vi "List Subscriptions.vi"(7 "Region":T1, 8 "error in (no error)":errorcluster, 11 "AWS Credentials":T2) -> (0 "error out":errorcluster, 3 "Subscriptions out":refnum<class "Subscription.lvclass">[](array[class]))   [LabVIEW 2015, in "NI_AWS_SNS.lvlib" / "Subscription.lvclass"]
uses:
  Subscription.lvclass
  Core/HTTP Request/AWS Credentials.ctl
  Core/HTTP Request/Region.ctl
  Core/HTTP Request/HTTP Request.lvclass/HTTP Request.ctl
  Core/HTTP Request/Write Credentials.vi
  Core/HTTP Request/Write Region.vi
  Core/HTTP Request/Write Service.vi
  Core/HTTP Request/Write Verify Server.vi
  Core/ARN/ARN.lvclass
  Core/HTTP Request/HTTP Request.lvclass
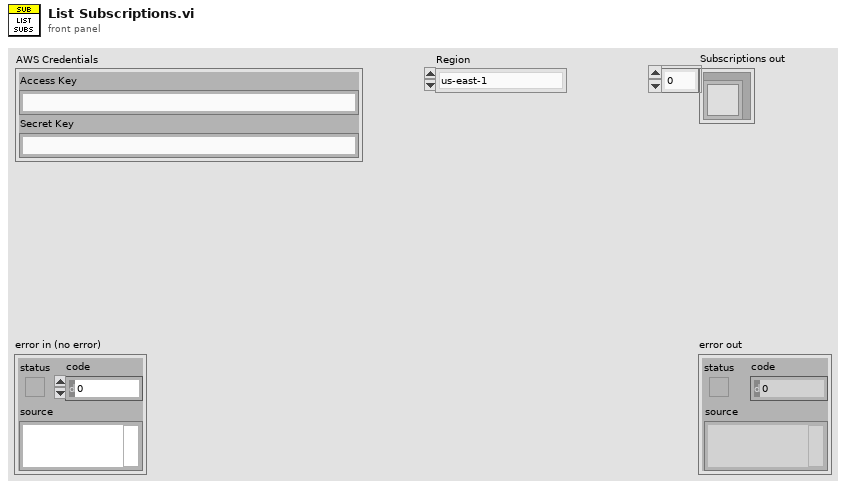
[diagram p1: front panel]
types:
  T1 = typedef "NI_AWS_Core.lvlib/HTTP Request.lvclass/Region.ctl" = enum16{"us-east-1", "us-east-2", "us-west-1", "us-west-2", "ap-northeast-1", "ap-northeast-2", "ap-southeast-1", "ap-southeast-2", "ca-central-1", "eu-central-1", "eu-west-1", "eu-west-2", "sa-east-1"}
  T2 = typedef "NI_AWS_Core.lvlib/HTTP Request.lvclass/AWS Credentials.ctl" = cluster{"Access Key":string, "Secret Key":string}
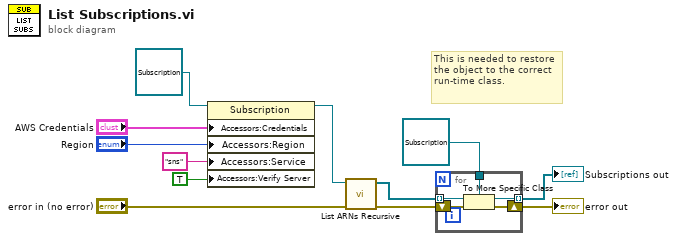
[diagram p0: block diagram]
diagram:
  # "This is needed to restore the object to the correct run-time class."
  n1 = property class="Subscription"(reference=refnum<class "Subscription.lvclass"> refnum ("NI_AWS_SNS.lvlib:Subscription"), "Accessors:Credentials"="AWS Credentials", "Accessors:Region"="Region", "Accessors:Service"="sns" ("Service"), "Accessors:Verify Server"=TRUE ("Verify Server")) -> (reference out=w10:refnum<class "Subscription.lvclass">)  [unwired: 1 in, 1 out]
  n2 = call "List ARNs Recursive.vi"("error in (no error)"="error in (no error)", "ARN in"=w10) -> ("error out"=w6:errorcluster, "ARNs out"=w8:refnum<class "ARN.lvclass">[])  [unwired: 8 in]
  n3 = for {
    tunnel: refnum<class "Subscription.lvclass"> refnum ("NI_AWS_SNS.lvlib:Subscription") -> [w17]
    tunnel: w8 -> [w16] mode=indexing
    tunnel: [w15] -> w4 mode=indexing
    shift-right: [w13] -> w1
    shift-left: w6 -> [w14]
    n4 = To More Specific Class(target class=w17, reference=w16, error in=w14) -> (specific class reference=w15:refnum<class "Subscription.lvclass">, error out=w13:errorcluster)
  }
  "error out" <- w1
  "Subscriptions out" <- w4
